vi "Binary_ConfusionMatrix.vi"(8 "error in (no error)":errorcluster, 9 "True Label":i32=1 caption="True Label (1)", 10 "Actual Labels":dbl[](array[numeric]), 11 "Predicted Labels":dbl[](array[numeric])) -> (0 "error out":errorcluster, 3 "Binary Confusion Matrix":T1)   [LabVIEW 2014]
uses:
  Controls/Binary_ConfusionMatrix.ctl
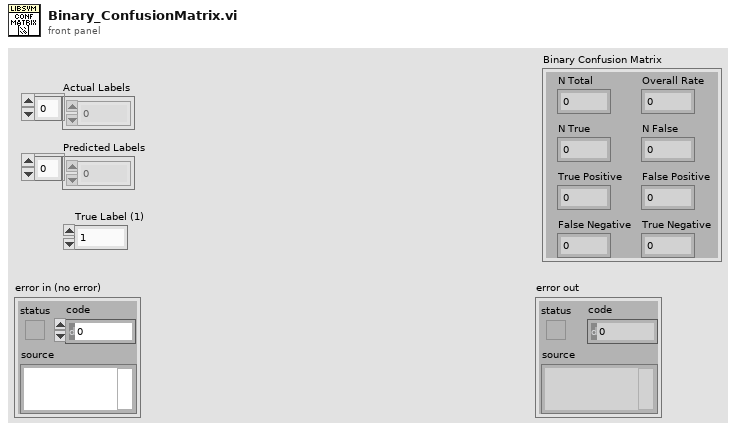
[diagram p1: front panel]
types:
  T1 = typedef "Binary_ConfusionMatrix.ctl" = cluster{"N Total":u32, "N True":u32, "N False":u32, "Overall Rate":dbl, "True Positive":dbl, "False Positive":dbl, "False Negative":dbl, "True Negative":dbl}
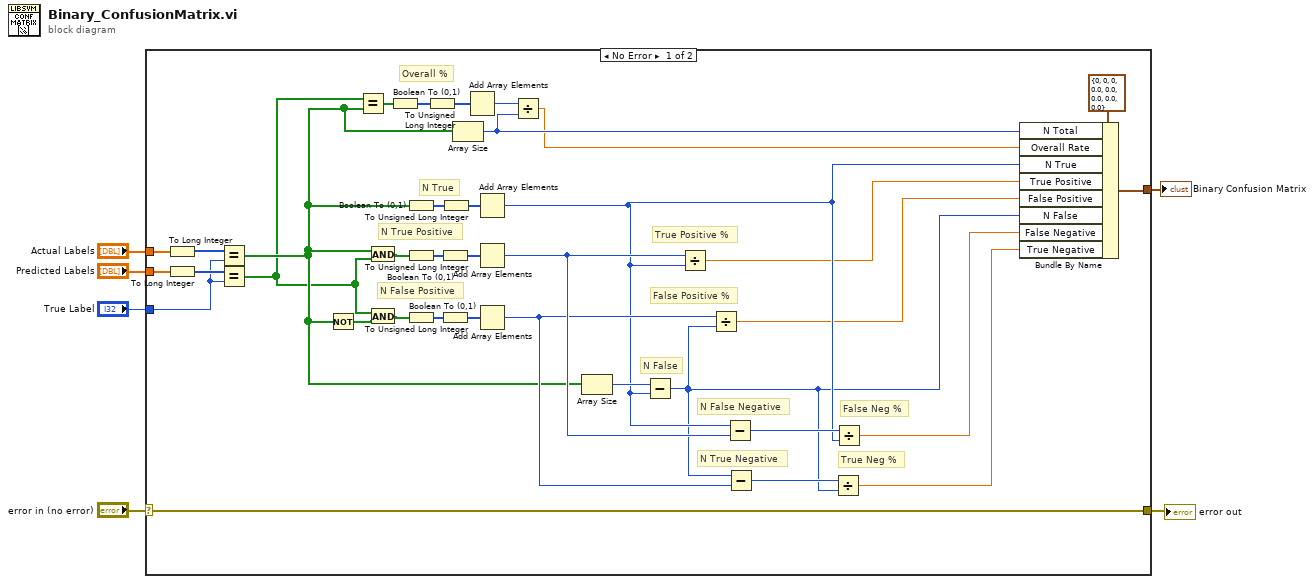
[diagram p0: block diagram]
diagram:
  n1 = case shown="No Error" "error in (no error)" {
    selector: "error in (no error)" -> [w7 w43]
    tunnel: [w7 w43] -> w6
    tunnel: "True Label" -> [w19 _]
    tunnel: "Actual Labels" -> [w23 _]
    tunnel: "Predicted Labels" -> [w22 _]
    tunnel: [w8 _] -> w1
    frame No Error {
      # "True Neg %"
      # "False Neg %"
      # "False Positive %"
      # "True Positive %"
      # "Overall %"
      # "N False Negative"
      # "N True Negative"
      # "N False"
      # "N False Positive"
      # "N True Positive"
      # "N True"
      n2 = To Long Integer(number=w23) -> (32bit integer=w21:i32[])
      n3 = To Long Integer(number=w22) -> (32bit integer=w20:i32[])
      n4 = Equal?(x=w21, y=w19) -> (x = y?=w18:bool[])
      n5 = Equal?(x=w20, y=w19) -> (x = y?=w17:bool[])
      n6 = Not(x=w18) -> (.not. x?=w34:bool[])
      n7 = Equal?(x=w17, y=w18) -> (x = y?=w31:bool[])
      n8 = And(x=w18, y=w17) -> (x .and. y?=w40:bool[])
      n9 = And(x=w17, y=w34) -> (x .and. y?=w35:bool[])
      n10 = Boolean To (0,1)(Boolean=w31) -> (0, 1=w32:i16[])
      n11 = Boolean To (0,1)(Boolean=w18) -> (0, 1=w42:i16[])
      n12 = Boolean To (0,1)(Boolean=w40) -> (0, 1=w39:i16[])
      n13 = Boolean To (0,1)(Boolean=w35) -> (0, 1=w36:i16[])
      n14 = To Unsigned Long Integer(number=w32) -> (unsigned 32bit integer=w30:u32[])
      n15 = To Unsigned Long Integer(number=w39) -> (unsigned 32bit integer=w38:u32[])
      n16 = To Unsigned Long Integer(number=w36) -> (unsigned 32bit integer=w37:u32[])
      n17 = To Unsigned Long Integer(number=w42) -> (unsigned 32bit integer=w41:u32[])
      n18 = Array Size(array=w18) -> (size(s)=w16:i32)
      n19 = Add Array Elements(numeric array=w30) -> (sum=w25:u32)
      n20 = Add Array Elements(numeric array=w41) -> (sum=w14:u32)
      n21 = Add Array Elements(numeric array=w38) -> (sum=w29:u32)
      n22 = Add Array Elements(numeric array=w37) -> (sum=w28:u32)
      n23 = Divide(x=w25, y=w16) -> (x/y=w15:dbl)
      n24 = Array Size(array=w18) -> (size(s)=w33:i32)
      n25 = Subtract(x=w33, y=w14) -> (x-y=w9:u32)
      n26 = Divide(x=w29, y=w14) -> (x/y=w13:dbl)
      n27 = Divide(x=w28, y=w9) -> (x/y=w12:dbl)
      n28 = Subtract(x=w14, y=w29) -> (x-y=w27:u32)
      n29 = Subtract(x=w9, y=w28) -> (x-y=w26:u32)
      n30 = Divide(x=w26, y=w9) -> (x/y=w10:dbl)
      n31 = Divide(x=w27, y=w14) -> (x/y=w11:dbl)
      n32 = Bundle By Name(cluster=T1 {"N Total"=0, "N True"=0, "N False"=0, "Overall Rate"=0.0, "True Positive"=0.0, "False Positive"=0.0, "False Negative"=0.0, "True Negative"=0.0} ("Binary Confusion Matrix"), "N Total"=w16, "Overall Rate"=w15, "N True"=w14, "True Positive"=w13, "False Positive"=w12, "N False"=w9, "False Negative"=w11, "True Negative"=w10) -> (w8:T1)
    }
    frame Error {
    }
  }
  "error out" <- w6
  "Binary Confusion Matrix" <- w1
